vi "Read Ack.vi"(7 "timeout in ms (-1)":i32=-1, 9 "ack id (0)":u32, 10 "channel":T1) -> (5 "timed out?":bool)   [LabVIEW 2019, in "MessengerM.lvlib"]
doc: "Waits for an acknowledgement from a Messenger channel. If no acknowledgement from the channel, this endpoint waits until the acknowledgement is available."
uses:
  <resource>/Channels/MessengerM/MessengerM.lvlib
  <resource>/Channels/MessengerM/))Channel.ctl
  <resource>/Channels/MessengerM/Element.ctl
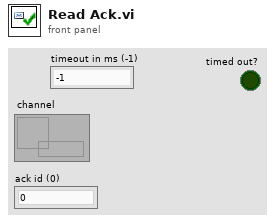
[diagram p1: front panel]
types:
  T1 = typedef "MessengerM.lvlib/))Channel.ctl" = refnum<queue>
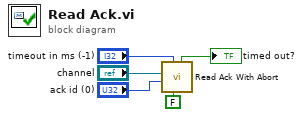
[diagram p0: block diagram]
diagram:
  n1 = call <resource>:"Read Ack With Abort.vi"("abort (F)"=FALSE, "timeout in ms (-1)"="timeout in ms (-1)", "ack id (0)"="ack id (0)", "channel"="channel") -> ("timed out?"=→"timed out?":bool)  [unwired: 6 in, 1 out]
